vi "XYStage.KIM101.SetResource.vi"(8 "error in (no error)":errorcluster, 10 "Resource":T1={"KCubeInertialMotorControl"=refnum, "Device"=refnum, "X Axis Channel"=1, "Y Axis Channel"=2} {"Y Axis Channel" items=["Channel1"=1, "Channel2"=2, "Channel3"=3, "Channel4"=4]; "X Axis Channel" items=["Channel1"=1, "Channel2"=2, "Channel3"=3, "Channel4"=4]}, 11 "XYStage.KIM101 in":refnum<class "XYStage.KIM101.lvclass">) -> (0 "error out":errorcluster, 3 "XYStage.KIM101 out":refnum<class "XYStage.KIM101.lvclass">)   [LabVIEW 2017, in "XYStage.KIM101.lvclass"]
uses:
  XYStage.KIM101.lvclass
  Typedefs/Resource--Cluster.ctl
  D:/upwork/Laser Measurement Tool/Laser/project/data/Thorlabs.MotionControl.Controls.dll
  data/Thorlabs.MotionControl.Controls.dll
  D:/upwork/Laser Measurement Tool/Laser/project/data/Thorlabs.MotionControl.KCube.InertialMotorCLI.dll
  data/Thorlabs.MotionControl.KCube.InertialMotorCLI.dll
  XYStage.KIM101.lvclass/XYStage.KIM101.ctl
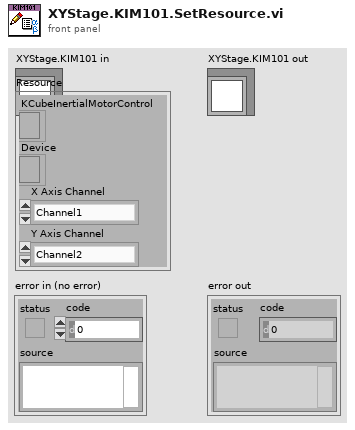
[diagram p1: front panel]
types:
  T1 = typedef "XYStage.KIM101.lvclass/Resource--Cluster.ctl" = cluster{"KCubeInertialMotorControl":refnum<k24>, "Device":refnum<k24>, "X Axis Channel":i32, "Y Axis Channel":i32}
  T2 = typedef "XYStage.KIM101.lvclass/PrivateData--Ref.ctl" = refnum<data-value>
  T3 = typedef "XYStage.KIM101.lvclass/PrivateData--Cluster.ctl" = cluster{"Resource":T1}
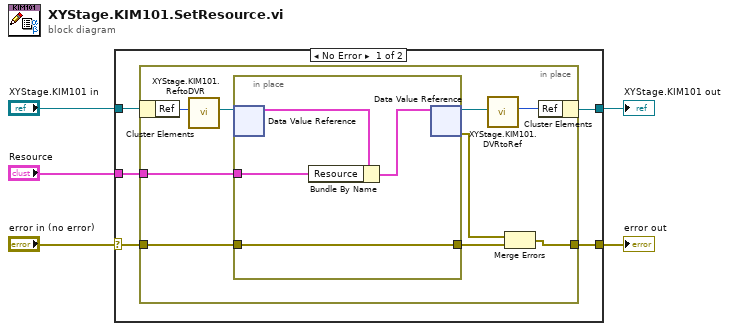
[diagram p0: block diagram]
diagram:
  n1 = case shown="No Error" "error in (no error)" {
    selector: "error in (no error)" -> [w7 w25]
    tunnel: [w6 w25] -> w4
    tunnel: [w9 w24] -> w2
    tunnel: "XYStage.KIM101 in" -> [w10 w24]
    tunnel: "Resource" -> [w8 _]
    frame No Error {
      n2 = in-place {
        in-place-border: w8 -> [w16]
        in-place-border: w7 -> [w13]
        in-place-border: [w11] -> w6
        n3 = in-place-cluster #1(w10) -> ("Ref"=w19:u32)
        n4 = call "XYStage.KIM101.ReftoDVR.vi"("Ref"=w19) -> ("Ref"=w17:T2)  [unwired: 10 in]
        n5 = in-place {
          in-place-border: w16 -> [w22]
          in-place-border: [w20] -> w12
          in-place-border: w13 -> [w20]
          n6 = in-place-dvr #2(w17) -> (w23:T3)  [unwired: 1 out]
          n7 = Bundle By Name(cluster=w23, "Resource"=w22) -> (w21:T3)
          n8 = in-place-dvr #2(w21) -> (w15:T2, w14:errorcluster)
        }
        n9 = call "XYStage.KIM101.DVRtoRef.vi"("Ref"=w15) -> ("Ref"=w18:u32)  [unwired: 10 in]
        n10 = Merge Errors(w14, w12) -> (w11:errorcluster)
        n11 = in-place-cluster #1("Ref"=w18) -> (w9:refnum<class "XYStage.KIM101.lvclass">)
      }
    }
    frame Error {
    }
  }
  "error out" <- w4
  "XYStage.KIM101 out" <- w2
